vi "MU set Calibration.vi"(8 "error in (no error)":errorcluster, 10 "CalibrationHandle":T1, 11 "MUhandle":u64) -> (0 "error out":errorcluster, 3 "function return":u32)   [LabVIEW 2017, in "MU_3SL_interface.lvlib"]
doc: "MU_PUBLIC MU_Error MU_setCalibration(MU_Handle handle, const MU_Calibration* calibration);"
uses:
  MU_3SL_interface.lvlib
  handles/CalibrationHandle.ctl
  lib/MU_3SL_interface.dll
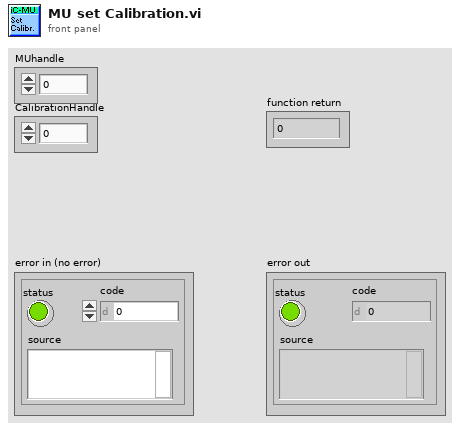
[diagram p1: front panel]
types:
  T1 = typedef "MU_3SL_interface.lvlib/CalibrationHandle.ctl" = u64
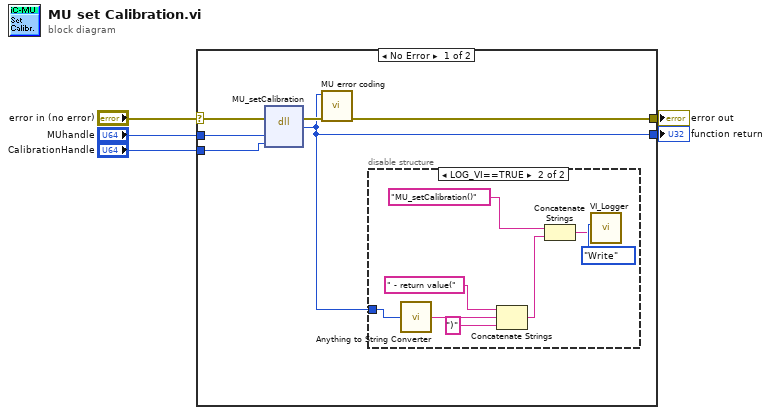
[diagram p0: block diagram]
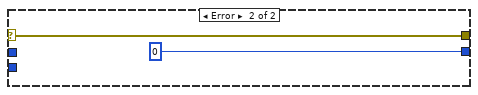
[diagram p3: hidden frame]
diagram:
  n1 = case shown="No Error" "error in (no error)" {
    selector: "error in (no error)" -> [w9 w21]
    tunnel: [w7 u32 0 ("return type")] -> w5
    tunnel: [w10 w21] -> w4
    tunnel: "CalibrationHandle" -> [w6 _]
    tunnel: "MUhandle" -> [w8 _]
    frame No Error {
      n2 = dll-call lib="C:/Users/bes/AppData/Roaming/work/mu_9so/icsubmodules/soft_mu_3sl_master/lv_interface/lib/MU_3SL_interface**.*" fn="MU_setCalibration"(error in=w9, "MUhandle"=w8, "CalibrationHandle"=w6) -> (error out=w11:errorcluster, "return type"=w7:u32)  [unwired: 4 in, 1 out]
      n3 = call "MU error coding.vi"("error in (no error)"=w11, "function return in"=w7) -> ("error out"=w10:errorcluster)  [unwired: 9 in]
      n4 = disable-structure shown="LOG_VI==TRUE" {
        disable-tunnel: w7 -> [_ w15]
        frame condition #0 {
        }
        frame condition #1 (active) {
          n5 = call "Anything to String Converter.vi"("anything"=w15) -> ("String"=w14:string)
          n6 = Concatenate Strings(" - return value(" ("string"), w14, ")" ("string")) -> (w12:string)
          n7 = Concatenate Strings("MU_setCalibration()" ("Info in"), w12) -> (w17:string)
          n8 = call "VI_Logger.vi"("Action (Read)"=enum16{"Write", "Read"}."Write", "Info in"=w17) -> ()  [unwired: 8 in, 2 out]
        }
      }
    }
    frame Error {
    }
  }
  "function return" <- w5
  "error out" <- w4
